vi "Get Configured Audio Devices.vi"(8 "error in (no error)":errorcluster) -> (0 "error out":errorcluster, 1 "Loopback Device Refnums":T1[](array[typedef]), 2 "Capture Device Refnums":T1[](array[typedef]), 3 "Playback Device Refnums":T1[](array[typedef]))   [LabVIEW 2020, in "G-Audio.lvlib"]
doc: "Get the references to all configured audio devices."
uses:
  G-Audio.lvlib
  Controls/Audio Device Refnum.ctl
  <vilib>/Utility/error.llb/Error Cluster From Error Code.vi
  lib/g_audio_32.dll
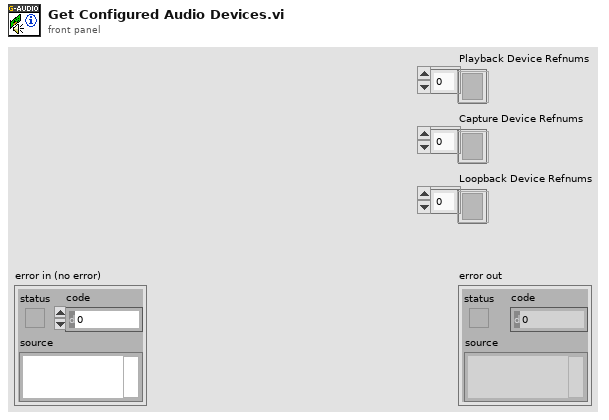
[diagram p1: front panel]
types:
  T1 = typedef "G-Audio.lvlib/Audio Device Refnum.ctl" = refnum<file>
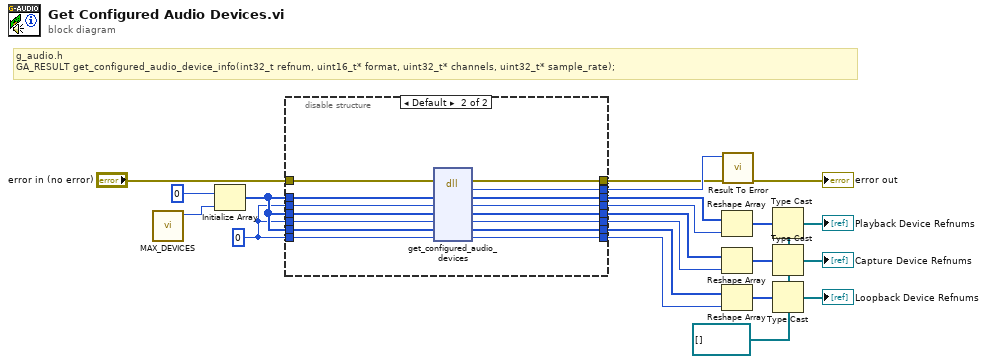
[diagram p0: block diagram]
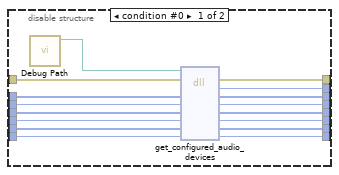
[diagram p2: hidden frame]
diagram:
  w10 = 0
  w3 = T1[] [] ("Audio Device Refnums")
  # "g_audio.h\nGA_RESULT get_configured_audio_device_info(int32_t refnum, uint16_t* format, uint32_t* channels, uint32_t* sample_rate);"
  n1 = call "MAX_DEVICES.vi"() -> ("MAX_DEVICES"=w17:i32)  [unwired: 11 in]
  n2 = Initialize Array(0, w17) -> (w11:i32[])
  n3 = disable-structure shown="Default" {
    disable-tunnel: "error in (no error)" -> [w37 w52]
    disable-tunnel: [w34 w50] -> w20
    disable-tunnel: [w36 w51] -> w19
    disable-tunnel: w11 -> [w35 w49]
    disable-tunnel: w10 -> [w32 w46]
    disable-tunnel: [w30 w48] -> w15
    disable-tunnel: [w31 w47] -> w12
    disable-tunnel: w11 -> [w29 w45]
    disable-tunnel: w11 -> [w27 w44]
    disable-tunnel: w10 -> [w28 w43]
    disable-tunnel: w10 -> [w26 w42]
    disable-tunnel: [w22 w41] -> w9
    disable-tunnel: [w23 w40] -> w8
    disable-tunnel: [w24 w39] -> w7
    disable-tunnel: [w25 w38] -> w6
    frame condition #0 {
      n4 = call "Debug Path.vi"() -> ("Debug Path"=w33:path)  [unwired: 11 in]
      n5 = dll-call lib="?" fn="get_configured_audio_devices"(path in=w33, error in=w37, "playback_refnums"=w35, "num_playback_refnums"=w32, "capture_refnums"=w29, "num_capture_refnums"=w28, "loopback_refnums"=w27, "num_loopback_refnums"=w26) -> (error out=w36:errorcluster, "result"=w34:i32, "playback_refnums"=w30:i32[], "num_playback_refnums"=w31:i32, "capture_refnums"=w22:i32[], "num_capture_refnums"=w23:i32, "loopback_refnums"=w24:i32[], "num_loopback_refnums"=w25:i32)  [unwired: 1 in, 1 out]
    }
    frame condition #1 (active) {
      n6 = dll-call lib="C:/github/dataflowg/g-audio/src/LabVIEW/G-Audio/lib/g_audio_*.*" fn="get_configured_audio_devices"(error in=w52, "playback_refnums"=w49, "num_playback_refnums"=w46, "capture_refnums"=w45, "num_capture_refnums"=w43, "loopback_refnums"=w44, "num_loopback_refnums"=w42) -> (error out=w51:errorcluster, "result"=w50:i32, "playback_refnums"=w48:i32[], "num_playback_refnums"=w47:i32, "capture_refnums"=w41:i32[], "num_capture_refnums"=w40:i32, "loopback_refnums"=w39:i32[], "num_loopback_refnums"=w38:i32)  [unwired: 2 in, 1 out]
    }
  }
  n7 = Reshape Array(w15, w12) -> (w13:i32[])
  n8 = Reshape Array(w9, w8) -> (w5:i32[])
  n9 = Reshape Array(w7, w6) -> (w4:i32[])
  n10 = call "Result To Error.vi"("error in (no error)"=w19, "Result Code"=w20) -> ("error out"=→"error out":errorcluster)  [unwired: 9 in]
  n11 = Type Cast(type=w3, x=w13) -> (*(type *) &x=→"Playback Device Refnums":T1[])
  n12 = Type Cast(type=w3, x=w5) -> (*(type *) &x=→"Capture Device Refnums":T1[])
  n13 = Type Cast(type=w3, x=w4) -> (*(type *) &x=→"Loopback Device Refnums":T1[])
